vi "Drive Code.vi"() -> ()   [LabVIEW 2012]
uses:
  <vilib>/Rock Robotics/WPI/Joystick/WPI_JoystickGetSetRefNum.vi
  Robot Global Data.vi
  Globals/Useful Values.vi
panel:
  out "Gyro?":bool
  out "axis 3 (throttle)":dbl
  out "axis 4":dbl
  in  "Gyro":dbl=-0.025
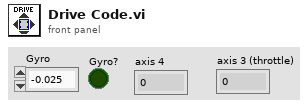
[diagram p1: front panel]
types:
  T1 = typedef "WPI_JoystickDevRef.ctl" = cluster{"Device":T2}
  T2 = typedef "WPI_JoystickDeviceEnum.ctl" = enum16{"USB 1", "USB 2", "USB 3", "USB 4", "Kinect 1", "Kinect 2"}
  T3 = typedef "WPI_MotorControlDeviceRef.ctl" = cluster{"DeviceStatus":errorcluster, "Type":enum16{"PWM", "CAN"}, "PWM":cluster{"Digital Module":T4, "PWM Channel":T5, "DeadBand":T6}, "CAN":cluster{"Device Number":u8, "Control Mode":T7, "Semaphore":T8, "Max Vout":dbl}, "Invert":bool, "TransformRef":T9, "InvTransformRef":T9}
  T4 = typedef "FPGA_TypedefDigitalModule.ctl" = enum16{"Digital Module 1", "Digital Module 2"}
  T5 = typedef "FPGA_DIOPWMChannel.ctl" = enum8{"PWM 1", "PWM 2", "PWM 3", "PWM 4", "PWM 5", "PWM 6", "PWM 7", "PWM 8", "PWM 9", "PWM 10", "Invalid"}
  T6 = typedef "WPI_PWMDeadband.ctl" = cluster{"Name":string, "maxPositivePwm":i32, "minPositivePwm":i32, "centerPwm":i32, "maxNegativePwm":i32, "minNegativePwm":i32, "angularRange":u16}
  T7 = typedef "WPI_CANJaguar_ControlMode.ctl" = enum8{"Percent VBus", "Current", "Speed", "Position", "Voltage"}
  T8 = typedef "Semaphore RefNum" = refnum<k1>
  T9 = typedef "WPI_PWMTransform_ConPane.ctl" = refnum<vi>
  T10 = typedef "WPI_JoystickButtonState.ctl" = cluster{"Button 1":bool, "Button 2":bool, "Button 3":bool, "Button 4":bool, "Button 5":bool, "Button 6":bool, "Button 7":bool, "Button 8":bool, "Button 9":bool, "Button 10":bool, "Button 11":bool, "Button 12":bool}
  T11 = typedef "WPI_GyroDevRef.ctl" = cluster{"DevStatus":errorcluster, "Analog Module":T12, "Analog Channel":T13, "Offset":dbl, "Gain (VoltsPerDegree/Second)":dbl}
  T12 = typedef "FPGA_TypedefAnalogModule.ctl" = enum16{"Analog Module 1", "Analog Module 2"}
  T13 = typedef "FPGA_AIChannel.ctl" = enum8{"AI 1", "AI 2", "AI 3", "AI 4", "AI 5", "AI 6", "AI 7", "AI 8", "Invalid"}
  T14 = typedef "WPI_DriverStationRobotMode2.ctl" = enum16{"Autonomous Disabled", "Autonomous Enabled", "Teleop Disabled", "Teleop Enabled", "Timeout", "Finish", "Test Disabled", "Test Enabled"}
  T15 = cluster{"axis 1 (x)":dbl, "axis 2 (y)":dbl, "axis 3 (throttle)":dbl, "axis 4":dbl, "axis 5":dbl, "axis 6":dbl}
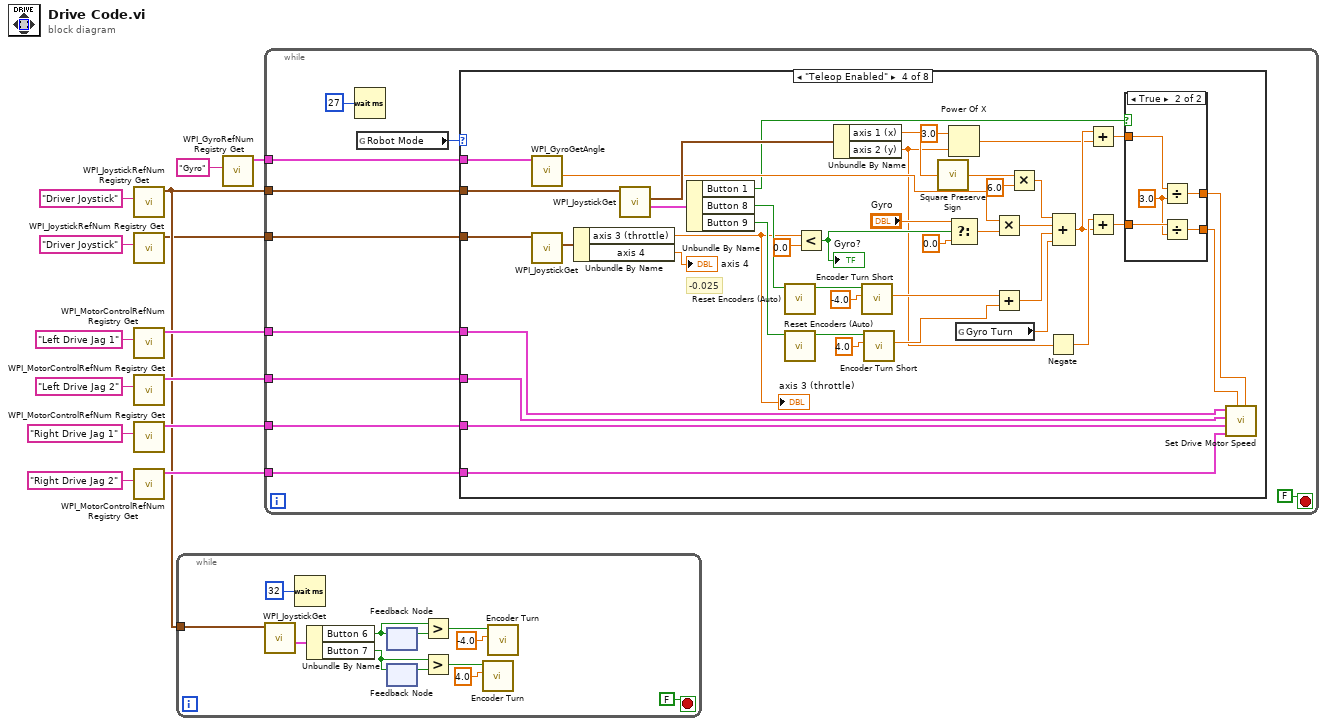
[diagram p0: block diagram]
diagram:
  n1 = call <vilib>:"WPI_JoystickRefNum Registry Get.vi"("refnum name"="Driver Joystick") -> ("JoystickDevRef"=w3:T1)  [unwired: 9 in, 1 out]
  n2 = call <vilib>:"WPI_JoystickRefNum Registry Get.vi"("refnum name"="Driver Joystick") -> ("JoystickDevRef"=w1:T1)  [unwired: 9 in, 1 out]
  n3 = call <vilib>:"WPI_MotorControlRefNum Registry Get.vi"("refnum name"="Left Drive Jag 1") -> ("MotorControlDevRef"=w4:T3)  [unwired: 9 in, 1 out]
  n4 = call <vilib>:"WPI_MotorControlRefNum Registry Get.vi"("refnum name"="Left Drive Jag 2") -> ("MotorControlDevRef"=w7:T3)  [unwired: 9 in, 1 out]
  n5 = call <vilib>:"WPI_MotorControlRefNum Registry Get.vi"("refnum name"="Right Drive Jag 1") -> ("MotorControlDevRef"=w5:T3)  [unwired: 9 in, 1 out]
  n6 = call <vilib>:"WPI_MotorControlRefNum Registry Get.vi"("refnum name"="Right Drive Jag 2") -> ("MotorControlDevRef"=w6:T3)  [unwired: 9 in, 1 out]
  n7 = while {
    tunnel: w3 -> [w25]
    stop <- FALSE stop-if-true
    n8 = call <vilib>:"WPI_JoystickGet.vi"("JoystickDevRef"=w25) -> ("Buttons"=w26:T10)  [unwired: 1 in, 5 out]
    n9 = Wait (ms)(milliseconds to wait=u32 32) -> ()  [unwired: 1 out]
    n10 = Unbundle By Name(w26) -> ("Button 6"=w18:bool, "Button 7"=w23:bool)
    n11 = feedback #1() -> (w17:bool)  [unwired: 1 in]
    n12 = feedback-in #1(w18) -> ()
    n13 = feedback #2() -> (w24:bool)  [unwired: 1 in]
    n14 = feedback-in #2(w23) -> ()
    n15 = Greater?(x=w18, y=w17) -> (0:w16:bool)
    n16 = Greater?(x=w23, y=w24) -> (0:w20:bool)
    n17 = call "Encoder Turn.vi"("Setpoint"=4.0, "Execute?"=w20) -> ()  [unwired: 9 in, 1 out]
    n18 = call "Encoder Turn.vi"("Setpoint"=-4.0, "Execute?"=w16) -> ()  [unwired: 9 in, 1 out]
  }
  n19 = call <vilib>:"WPI_GyroRefNum Registry Get.vi"("refnum name"="Gyro") -> ("GyroDevRef"=w9:T11)  [unwired: 9 in, 1 out]
  n20 = while {
    tunnel: w3 -> [w34]
    tunnel: w9 -> [w33]
    tunnel: w7 -> [w31]
    tunnel: w6 -> [w30]
    tunnel: w5 -> [w29]
    tunnel: w4 -> [w28]
    tunnel: w1 -> [w27]
    stop <- FALSE stop-if-true
    n21 = Wait (ms)(milliseconds to wait=u32 27) -> ()  [unwired: 1 out]
    n22 = global read "Robot Global Data.vi" "Robot Mode"() -> (w35:T14)
    n23 = case shown="\"Teleop Enabled\"" w35 {
      tunnel: w34 -> [_ _ _ w72 _ _ _ _]
      tunnel: w33 -> [_ _ _ w71 _ _ _ _]
      tunnel: w31 -> [_ _ _ w65 _ _ _ _]
      tunnel: w30 -> [_ _ _ w68 _ _ _ _]
      tunnel: w29 -> [_ _ _ w67 _ _ _ _]
      tunnel: w28 -> [_ _ _ w66 _ _ _ _]
      tunnel: w27 -> [_ _ _ w46 _ _ _ _]
      frame "Autonomous Disabled", Default {
      }
      frame "Autonomous Enabled" {
      }
      frame "Teleop Disabled" {
      }
      frame "Teleop Enabled" {
        # "-0.025"
        n24 = call <vilib>:"WPI_GyroGetAngle.vi"("GyroDevRef"=w71) -> ("Angular Rate"=w78:dbl)  [unwired: 7 in, 3 out]
        n25 = call <vilib>:"WPI_JoystickGet.vi"("JoystickDevRef"=w46) -> ("Axes"=w45:T15)  [unwired: 1 in, 5 out]
        n26 = Unbundle By Name(w45) -> ("axis 3 (throttle)"=w39:dbl, "axis 4"=→"axis 4":dbl)
        "axis 3 (throttle)" <- w39
        n27 = call <vilib>:"WPI_JoystickGet.vi"("JoystickDevRef"=w72) -> ("Buttons"=w77:T10, "Axes"=w79:T15)  [unwired: 1 in, 4 out]
        n28 = Unbundle By Name(w77) -> ("Button 1"=w74:bool, "Button 8"=w57:bool, "Button 9"=w56:bool)
        n29 = call "Reset Encoders (Auto).vi"("Execute?"=w57) -> ("Done"=w63:bool)  [unwired: 10 in]
        n30 = call "Reset Encoders (Auto).vi"("Execute?"=w56) -> ("Done"=w62:bool)  [unwired: 10 in]
        n31 = Less?(x=w39, y=0.0) -> (x < y?=w47:bool)
        "Gyro?" <- w47
        n32 = Unbundle By Name(w79) -> ("axis 1 (x)"=w38:dbl, "axis 2 (y)"=w37:dbl)
        n33 = call "Encoder Turn Short.vi"("Setpoint"=-4.0, "Execute?"=w63) -> ("output"=w59:dbl)  [unwired: 8 in, 1 out]
        n34 = call "Encoder Turn Short.vi"("Setpoint"=4.0, "Execute?"=w62) -> ("output"=w58:dbl)  [unwired: 8 in, 1 out]
        n35 = call "Square Preserve Sign.vi"("In"=w38) -> ("Out"=w48:dbl)
        n36 = Power Of X(1:w37, 2:3.0 ("y")) -> (0:w49:dbl)
        n37 = Select(t="Gyro", s=w47, f=0.0) -> (s? t:f=w40:dbl)
        n38 = global read "Useful Values.vi" "Gyro Turn"() -> (w52:dbl)
        n39 = Multiply(x=w78, y=w40) -> (x*y=w54:dbl)
        n40 = Add(x=w59, y=w58) -> (x+y=w53:dbl)
        n41 = Multiply(x=w48, y=6.0) -> (x*y=w55:dbl)
        n42 = Negate(x=w37) -> (-x=w70:dbl)
        n43 = Compound Arithmetic op=ADD(w55, w54, w53, w52) -> (w51:dbl)
        n44 = Add(x=w51, y=w49) -> (x+y=w73:dbl)
        n45 = Add(x=w70, y=w51) -> (x+y=w76:dbl)
        n46 = case shown="True" w74 {
          tunnel: w76 -> [w81 w84]
          tunnel: w73 -> [w80 w83]
          tunnel: [w81 w85] -> w64
          tunnel: [w80 w86] -> w69
          frame False {
          }
          frame True {
            w82 = 3.0 ("y")
            n47 = Divide(x=w83, y=w82) -> (x/y=w86:dbl)
            n48 = Divide(x=w84, y=w82) -> (x/y=w85:dbl)
          }
        }
        n49 = call "Set Drive Motor Speed.vi"("Right Output"=w69, "Left Output"=w64, "Right Drive Jag 2"=w68, "Right Drive Jag 1"=w67, "Left Drive Jag 2"=w65, "Left Drive Jag 1"=w66) -> ()  [unwired: 6 in]
      }
      frame "Timeout" {
      }
      frame "Finish" {
      }
      frame "Test Disabled" {
      }
      frame "Test Enabled" {
      }
    }
  }
